vi "vipbBuild.vi"() -> (0 "error out":errorcluster)   [LabVIEW 2014, in "vipm-build-tools.lvlib"]
uses:
  vipm-build-tools.lvlib
  <vilib>/Wiresmith Technology/LabVIEW CLI/CLI Class/CLI.lvclass
  <vilib>/Utility/error.llb/DialogType.ctl
  <vilib>/JKI/VIPM API/VIPM API_vipm_api.lvlib
  build/lvcommonbuild.lvlib
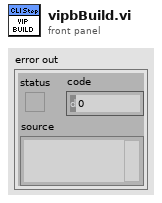
[diagram p1: front panel]
types:
  T1 = enum16{"open", "replace", "create", "open or create", "replace or create", "replace or create with confirmation"}
  T2 = typedef "DialogType.ctl" = u16
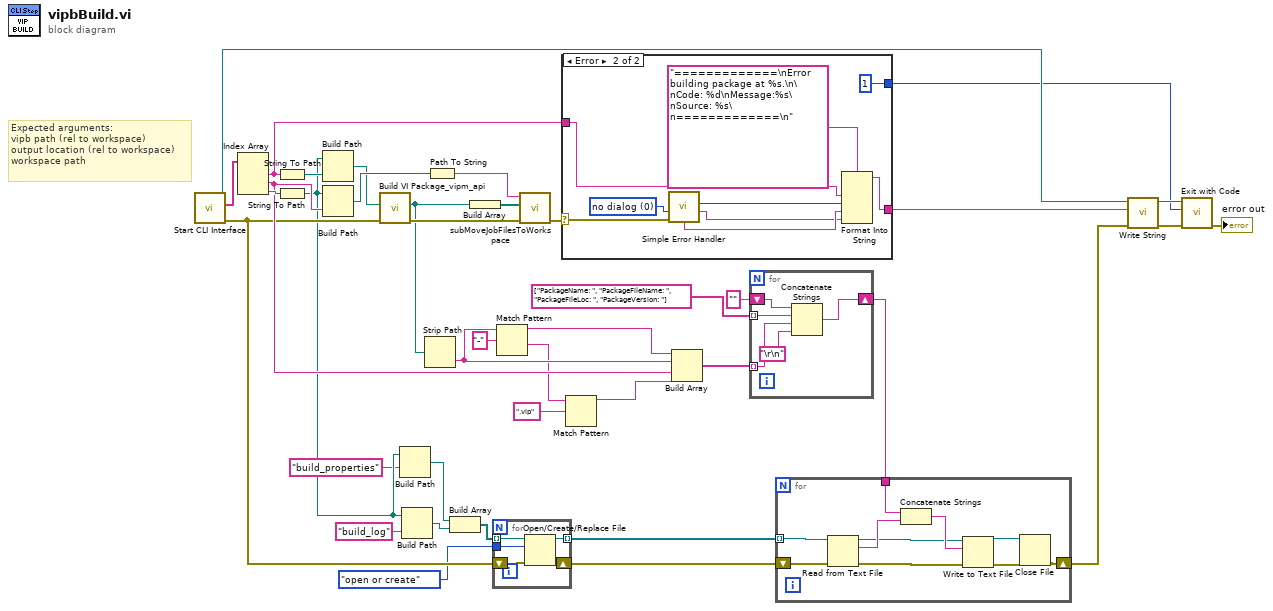
[diagram p0: block diagram]
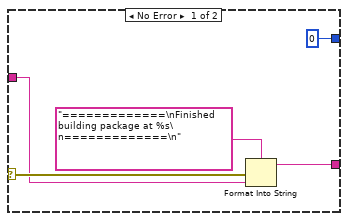
[diagram p2: hidden frame]
diagram:
  # "Expected arguments:\nvipb path (rel to workspace)\noutput location (rel to workspace)\nworkspace path"
  n1 = call <vilib>:"Start CLI Interface.vi"() -> ("error out"=w16:errorcluster, "Custom Parameters"=w39:string[], "CLI out"=w37:refnum<class "CLI.lvclass">)  [unwired: 9 in]
  n2 = Index Array(array=w39) -> (element #1=w19:string, element #2=w18:string, element #3=w31:string)  [unwired: 3 in]
  n3 = String To Path(string=w19) -> (path=w33:path)
  n4 = String To Path(string=w31) -> (path=w7:path)
  n5 = Build Path(base path=w7, name or relative path=w33) -> (appended path=w25:path)
  n6 = Build Path(base path=w7, name or relative path=w18) -> (appended path=w30:path)
  n7 = call <vilib>:"Build VI Package_vipm_api.vi"("error in (no error)"=w16, "Path to VIPB File"=w25) -> ("error out"=w29:errorcluster, "Build Output"=w23:path)  [unwired: 8 in]
  n8 = Build Path(base path=w7, name or relative path="build_properties") -> (appended path=w4:path)
  n9 = Build Path(base path=w7, name or relative path="build_log") -> (appended path=w3:path)
  n10 = Strip Path(path=w23) -> (name=w20:string)  [unwired: 1 out]
  n11 = Path To String(path=w30) -> (string=w27:string)
  n12 = Build Array(w4, w3) -> (w2:path[])
  n13 = Build Array(w23) -> (w26:path[])
  n14 = for {
    tunnel: w2 -> [w43] mode=indexing
    tunnel: T1."open or create" ("operation (0:open)") -> [w42]
    tunnel: [w41] -> w1 mode=indexing
    shift-right: [w40] -> w14
    shift-left: w16 -> [w44]
    n15 = Open/Create/Replace File(file path (use dialog)=w43, error in=w44, operation (0:open)=w42) -> (refnum out=w41:refnum<file>, error out=w40:errorcluster)  [unwired: 3 in, 1 out]
  }
  n16 = Match Pattern(string=w20, regular expression="-") -> (before substring=w21:string, after substring=w10:string)  [unwired: 1 in, 2 out]
  n17 = call "subMoveJobFilesToWorkspace.vi"("error in (no error)"=w29, "Generated Files"=w26, "Workspace Path"=w27) -> ("error out"=w28:errorcluster)  [unwired: 8 in]
  n18 = case shown="Error" w28 {
    selector: w28 -> [w48 w57]
    tunnel: w19 -> [w47 w53]
    tunnel: [w46 w58] -> w38
    tunnel: [0 ("Exit Code (0)") 1 ("Exit Code (0)")] -> w34
    frame No Error {
      n19 = Format Into String(format string="=============\nFinished building package at %s\n=============\n", error in=w48, w47) -> (resulting string=w46:string)  [unwired: 1 in, 1 out]
    }
    frame Error {
      w56 = T2 0 items=["no dialog", "OK message", "continue or stop message", "OK message + warnings", "continue/stop + warnings"] ("type of dialog (OK msg:1)")
      n20 = call <vilib>:"Simple Error Handler.vi"("type of dialog (OK msg:1)"=w56, "error in (no error)"=w57) -> ("code out"=w50:i32, "source out"=w51:string, "message"=w52:string)  [unwired: 3 in, 2 out]
      n21 = Format Into String(format string="=============\nError building package at %s.\n\nCode: %d\nMessage:%s\nSource: %s\n=============\n", w53, w50, w52, w51) -> (resulting string=w58:string)  [unwired: 2 in, 1 out]
    }
  }
  n22 = Match Pattern(string=w10, regular expression=".vip") -> (before substring=w8:string)  [unwired: 1 in, 3 out]
  n23 = Build Array(w21, w20, w18, w8) -> (w17:string[])
  n24 = for {
    tunnel: string[] ["PackageName: ", "PackageFileName: ", "PackageFileLoc: ", "PackageVersion: "] -> [w63] mode=indexing
    tunnel: w17 -> [w62] mode=indexing
    shift-right: [w60] -> w12
    shift-left: "" -> [w59]
    n25 = Concatenate Strings(w59, w63, w62, "\r\n") -> (w60:string)
  }
  n26 = for {
    tunnel: w12 -> [w72]
    shift-right: [w65] -> w11
    shift-left: w14 -> [w73]
    tunnel: w1 -> [w64] mode=indexing
    n27 = Read from Text File(file (use dialog)=w64, error in=w73) -> (refnum out=w69:refnum<file>, text=w71:string, error out=w68:errorcluster)  [unwired: 2 in, 1 out]
    n28 = Concatenate Strings(w72, w71) -> (w70:string)
    n29 = Write to Text File(file (use dialog)=w69, text=w70, error in=w68) -> (refnum out=w67:refnum<file>, error out=w66:errorcluster)  [unwired: 1 in, 1 out]
    n30 = Close File(refnum=w67, error in=w66) -> (error out=w65:errorcluster)  [unwired: 1 out]
  }
  n31 = call <vilib>:"Write String.vi"("error in (no error)"=w11, "Text to Write"=w38, "CLI in"=w37) -> ("error out"=w36:errorcluster, "CLI out"=w35:refnum<class "CLI.lvclass">)  [unwired: 7 in]
  n32 = call <vilib>:"Exit with Code.vi"("error in (no error)"=w36, "Exit Code (0)"=w34, "CLI in"=w35) -> ("error out"=→"error out":errorcluster)  [unwired: 8 in]
